vi "adjust_position.vi"(9 "Y Offset":i32, 10 "X Offset":i32, 11 "Position In":cluster{"Left":i32, "Top":i32}) -> (3 "Position Out":cluster{"Left":i32, "Top":i32})   [LabVIEW 2018]
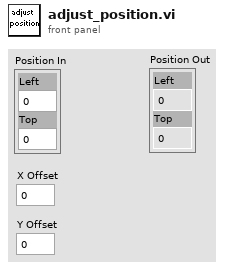
[diagram p1: front panel]
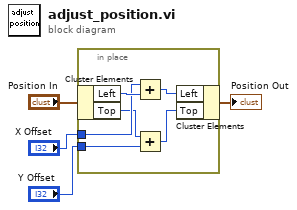
[diagram p0: block diagram]
diagram:
  n1 = in-place {
    in-place-border: "X Offset" -> [w9]
    in-place-border: "Y Offset" -> [w7]
    n2 = in-place-cluster #1("Position In") -> ("Left"=w10:i32, "Top"=w8:i32)
    n3 = Add(x=w9, y=w10) -> (x+y=w5:i32)
    n4 = Add(x=w8, y=w7) -> (x+y=w6:i32)
    n5 = in-place-cluster #1("Left"=w5, "Top"=w6) -> (→"Position Out":cluster{"Left":i32, "Top":i32})
  }
